vi "Add Time to Record.vi"(5 "Array Size (1)":i32=1, 7 "Nanosecond Counter":i64, 8 "error in (no error)":errorcluster, 9 "Time":dbl, 10 "Group Name":string, 11 "TDMS In":refnum<k34>) -> (0 "error out":errorcluster, 3 "TDMS Out":refnum<k34>)   [LabVIEW 2021]
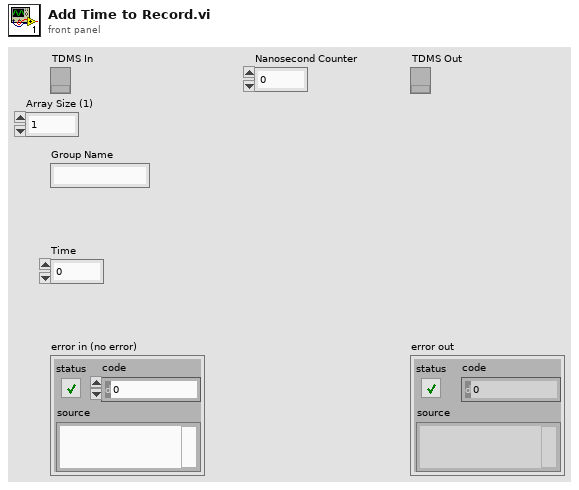
[diagram p1: front panel]
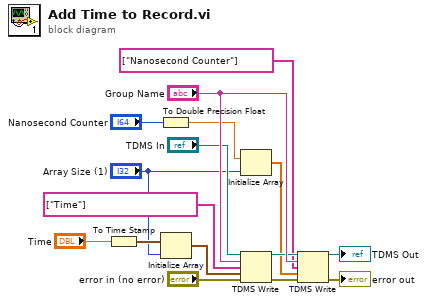
[diagram p0: block diagram]
diagram:
  n1 = To Time Stamp(1:"Time") -> (0:w5:timestamp)
  n2 = To Double Precision Float(number="Nanosecond Counter") -> (double precision float=w3:dbl)
  n3 = Initialize Array(w5, "Array Size (1)") -> (w4:timestamp[])
  n4 = Initialize Array(w3, "Array Size (1)") -> (w2:dbl[])
  n5 = TDMS Write(0:"TDMS In", 5:"Group Name", 7:string[] ["Time"] ("channel name(s) in (Untitled)"), 9:w4, 11:"error in (no error)") -> (4:w9:refnum<k34>, 15:w8:errorcluster)  [unwired: 1 in, 2 out]
  n6 = TDMS Write(0:w9, 5:"Group Name", 7:string[] ["Nanosecond Counter"] ("channel name(s) in (Untitled)"), 9:w2, 11:w8) -> (4:→"TDMS Out":refnum<k34>, 15:→"error out":errorcluster)  [unwired: 1 in, 2 out]
